vi "In_phase_Send.vi"() -> ()   [LabVIEW 2023]
uses:
  <vilib>/Utility/file.llb/Read Delimited Spreadsheet (string).vi
panel:
  out "Array":i32[](array[numeric])
  out "error out":errorcluster
  in  "CH ON/OFF":u16(ring) items=["ON", "OFF"]
  in  "Polarity":u16(ring) items=["V", "H"]
  in  "TRXmode":u16(ring)=1 items=["Rx"=2, "Tx"=1]
  in  "TCPIPin":T1={"address"="192.168.100.111", "remote port or service name"=5025, "timeout ms (60000)"=10000}
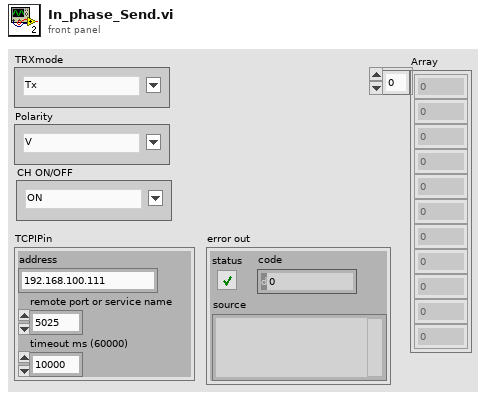
[diagram p1: front panel]
types:
  T1 = cluster{"address":string, "remote port or service name":u16, "timeout ms (60000)":i32}
  T2 = cluster{"Mode":u16, "Polarity":u16, "CH_ON/OFF":u16, "Channel":i32, "Gain":i32, "Phase":i32}
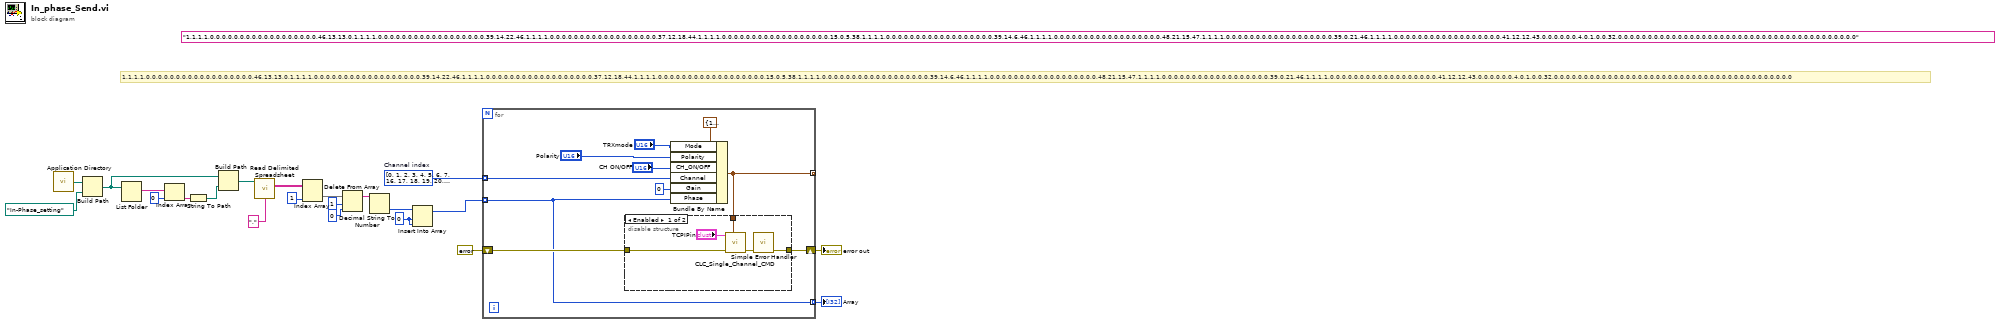
[diagram p0: block diagram]
diagram:
  (unwired) "1,1,1,1,0,0,0,0,0,0,0,0,0,0,0,0,0,0,0,0,0,0,46,13,13,0,1,1,1,1,0,0,0,0,0,0,0,0,0,0,0,0,0,0,0,0,0,0,39,14,22,46,1,1,1,1,0,0,0,0,0,0,0,0,0,0,0,0,0,0,0,0,0,0,37,12,18,44,1,1,1,1,0,0,0,0,0,0,0,0,0,0,0,0,0,0,0,0,0,0,15,0,5,38,1,1,1,1,0,0,0,0,0,0,0,0,0,0,0,0,0,0,0,0,0,0,39,14,6,46,1,1,1,1,0,0,0,0,0,0,0,0,0,0,0,0,0,0,0,0,0,0,48,21,15,47,1,1,1,1,0,0,0,0,0,0,0,0,0,0,0,0,0,0,0,0,0,0,39,0,21,46,1,1,1,1,0,0,0,0,0,0,0,0,0,0,0,0,0,0,0,0,0,0,41,12,12,43,0,0,0,0,0,0,4,0,1,0,0,32,0,0,0,0,0,0,0,0,0,0,0,0,0,0,0,0,0,0,0,0,0,0,0,0,0,0,0,0,0,0,0,0,0,0,0,0,0,0,0,0"
  w3 = i32[] [0, 1, 2, 3, 4, 5, 6, 7, 16, 17, 18, 19, 20, 21, 22, 23, 32, 33, 34, 35, 36, 37, 38, 39, 48, 49, 50, 51, 52, 53, 54, 55]  # Channel index
  w6 = 0 ("index")
  # "1,1,1,1,0,0,0,0,0,0,0,0,0,0,0,0,0,0,0,0,0,0,46,13,13,0,1,1,1,1,0,0,0,0,0,0,0,0,0,0,0,0,0,0,0,0,0,0,39,14,22,46,1,1,1,1,0,0,0,0,0,0,0,0,0,0,0,0,0,0,0,0,0,0,37,12,18,44,1,1,1,1,0,0,0,0,0,0,0,0,0,0,0,0,0,0,0,0,0,0,15,0,5,38,1,1,1,1,0,0,0,0,0,0,0,0,0,0,0,0,0,0,0,0,0,0,39,14,6,46,1,1,1,1,0,0,0,0,0,0,0,0,0,0,0,0,0,0,0,0,0,0,48,21,15,47,1,1,1,1,0,0,0,0,0,0,0,0,0,0,0,0,0,0,0,0,0,0,39,0,21,46,1,1,1,1,0,0,0,0,0,0,0,0,0,0,0,0,0,0,0,0,0,0,41,12,12,43,0,0,0,0,0,0,4,0,1,0,0,32,0,0,0,0,0,0,0,0,0,0,0,0,0,0,0,0,0,0,0,0,0,0,0,0,0,0,0,0,0,0,0,0,0,0,0,0,0,0,0,0"
  n1 = call <vilib>:"Application Directory.vi"() -> ("Application Directory"=w22:path)
  n2 = Build Path(base path=w22, name or relative path=path "In-Phase_setting") -> (appended path=w18:path)
  n3 = List Folder(path=w18) -> (filenames=w20:string[])  [unwired: 3 in, 3 out]
  n4 = Index Array(array=w20, index=0) -> (element=w17:string)
  n5 = String To Path(string=w17) -> (path=w16:path)
  n6 = Build Path(base path=w18, name or relative path=w16) -> (appended path=w15:path)
  n7 = call-poly <vilib>:"Read Delimited Spreadsheet.vi"("file path (dialog if empty)"=w15, "delimiter (\\t)"="," ("delimiter (\\t)")) -> ("all rows"=w13:string[][])  [unwired: 8 in, 5 out]
  n8 = Index Array(array=w13, index (col)=1 ("index (row)")) -> (element=w11:string[])  [unwired: 1 in]
  n9 = Delete From Array(array=w11, length=1, index=0) -> (array with subset deleted=w8:string[])  [unwired: 1 out]
  n10 = Decimal String To Number(string=w8) -> (number=w7:i32[])  [unwired: 2 in, 1 out]
  n11 = Insert Into Array(array=w7, index=w6, new element=w6) -> (w5:i32[])
  n12 = for {
    tunnel: w5 -> [w23] mode=indexing
    shift-right: [w31] -> w2
    shift-left: errorcluster {"status"=FALSE, "code"=0, "source"=""} ("error in") -> [w27]
    tunnel: w3 -> [w29] mode=indexing
    tunnel: [w28] -> _ mode=indexing
    tunnel: [w23] -> w1 mode=indexing
    n13 = Bundle By Name(cluster=T2 {"Mode"=1, "Polarity"=1, "CH_ON/OFF"=0, "Channel"=21, "Gain"=0, "Phase"=55} ("Channel params"), "Mode"="TRXmode", "Polarity"="Polarity", "CH_ON/OFF"="CH ON/OFF", "Channel"=w29, "Gain"=0, "Phase"=w23) -> (w28:T2)
    n14 = disable-structure shown="Enabled" {
      disable-tunnel: [w34 w38] -> w31
      disable-tunnel: w28 -> [w33 _]
      disable-tunnel: w27 -> [w36 w38]
      frame Enabled {
        n15 = call "CLC_Single_Channel_CMD.vi"("Channel params"=w33, "error in"=w36, "TCPIPin"="TCPIPin") -> ("error out"=w35:errorcluster)  [unwired: 6 in, 2 out]
        n16 = call <vilib>:"Simple Error Handler.vi"("error in (no error)"=w35) -> ("error out"=w34:errorcluster)  [unwired: 4 in, 4 out]
      }
      frame Disabled {
      }
    }
  }
  "error out" <- w2
  "Array" <- w1
